vi "get binary trace.vi"(7 "error in (no error)":errorcluster, 9 "Trace Name (0:Trace1)":u16(ring) items=["Trace1", "Trace2", "Trace3", "Trace4", "Trace5", "Trace6", "Line1", "Line2"], 10 "VISA resource in":refnum<visa-resource-name>) -> (0 "error out":errorcluster, 1 "Stop frequency(Hz)":dbl format="%#_13g", 2 "Start frequency (Hz)":dbl format="%#_13g", 3 "VISA resource out":refnum<visa-resource-name>, 4 "Number of points":i32, 5 "Linear frequecny increment (Hz)":dbl format="%#_13g", 6 "Trace Array (1D)":dbl[](array[numeric]))   [LabVIEW 2016]
doc: "Get binary trace information from PSA screen, output start/stop/frequency, linear frequency increment, Y value 1D Array data."
panel:
  out "Waveform Graph":dbl[](graph)
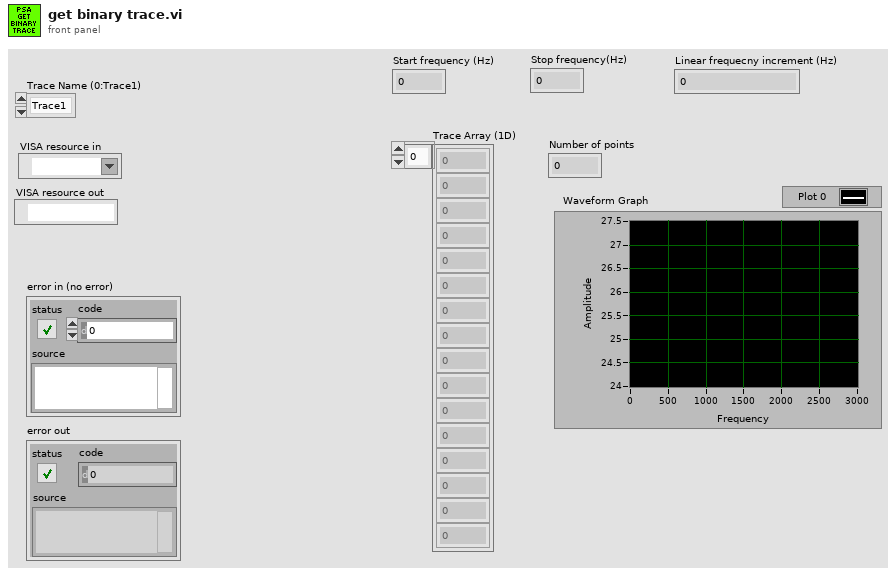
[diagram p1: front panel]
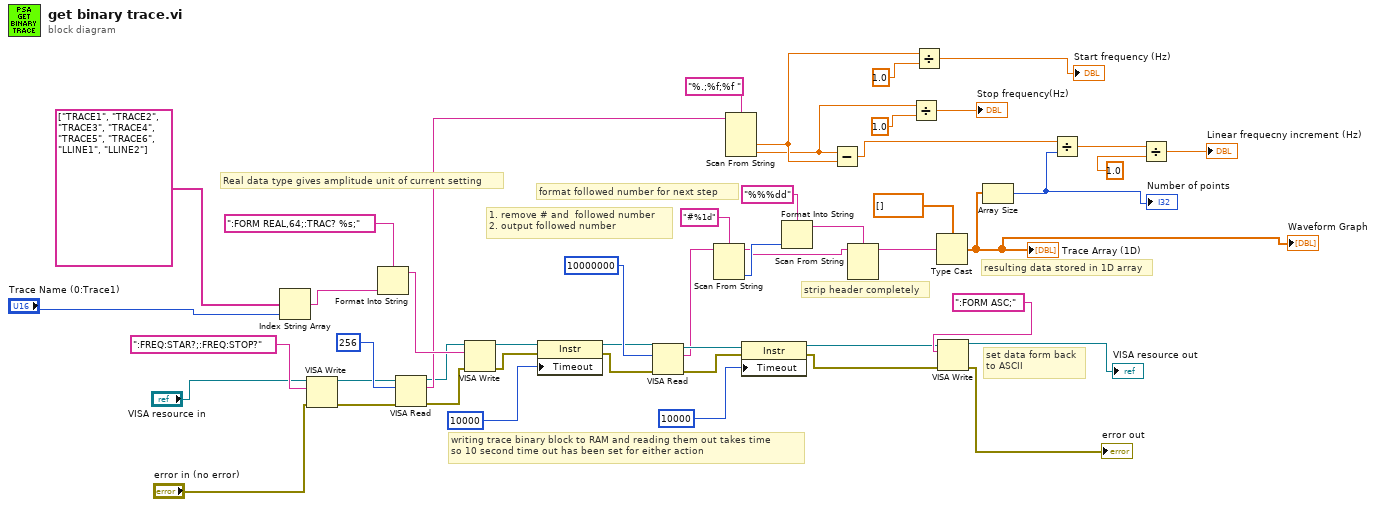
[diagram p0: block diagram]
diagram:
  # "set data form back\nto ASCII"
  # "writing trace binary block to RAM and reading them out takes time\nso 10 second time out has been set for either action"
  # "resulting data stored in 1D array"
  # "strip header completely"
  # "format followed number for next step"
  # "1. remove # and  followed number\n2. output followed number"
  # "Real data type gives amplitude unit of current setting"
  n1 = Index String Array(1:"Trace Name (0:Trace1)", 2:string[] ["TRACE1", "TRACE2", "TRACE3", "TRACE4", "TRACE5", "TRACE6", "LLINE1", "LLINE2"] ("string array")) -> (0:w46:string)  [unwired: 1 in]
  n2 = VISA Write(VISA resource name="VISA resource in", write buffer=":FREQ:STAR?;:FREQ:STOP?", error in (no error)="error in (no error)") -> (VISA resource name out=w27:refnum<visa-resource-name>, error out=w20:errorcluster)  [unwired: 1 out]
  n3 = Format Into String(format string=":FORM REAL,64;:TRAC? %s;", w46) -> (resulting string=w45:string)  [unwired: 2 in, 1 out]
  n4 = VISA Read(VISA resource name=w27, byte count=u32 256, error in (no error)=w20) -> (VISA resource name out=w12:refnum<visa-resource-name>, read buffer=w25:string, error out=w19:errorcluster)  [unwired: 1 out]
  n5 = VISA Write(VISA resource name=w12, write buffer=w45, error in (no error)=w19) -> (VISA resource name out=w43:refnum<visa-resource-name>, error out=w18:errorcluster)  [unwired: 1 out]
  n6 = property class="Instr"(reference=w43, error in=w18, "Timeout"=u32 10000 ("General Settings:Timeout Value")) -> (reference out=w41:refnum<visa-resource-name>, error out=w17:errorcluster)
  n7 = VISA Read(VISA resource name=w41, byte count=u32 10000000, error in (no error)=w17) -> (VISA resource name out=w39:refnum<visa-resource-name>, read buffer=w38:string, error out=w16:errorcluster)  [unwired: 1 out]
  n8 = Scan From String(format string="#%1d", input string=w38) -> (remaining string=w34:string, output 1=w36:i32)  [unwired: 3 in, 2 out]
  n9 = Scan From String(format string="%.;%f;%f ", input string=w25) -> (output 1=w11:dbl, output 2=w9:dbl)  [unwired: 4 in, 3 out]
  n10 = property class="Instr"(reference=w39, error in=w16, "Timeout"=u32 10000 ("General Settings:Timeout Value")) -> (reference out=w22:refnum<visa-resource-name>, error out=w15:errorcluster)
  n11 = Format Into String(format string="%%%dd", w36) -> (resulting string=w33:string)  [unwired: 2 in, 1 out]
  n12 = Subtract(x=w9, y=w11) -> (x-y=w24:dbl)
  n13 = Scan From String(format string=w33, input string=w34) -> (remaining string=w32:string)  [unwired: 4 in, 2 out]
  n14 = Divide(x=w9, y=1.0) -> (x/y=→"Stop frequency(Hz)":dbl)
  n15 = Divide(x=w11, y=1.0) -> (x/y=→"Start frequency (Hz)":dbl)
  n16 = Type Cast(type=dbl[] [], x=w32) -> (*(type *) &x=w1:dbl[])
  "Trace Array (1D)" <- w1
  "Waveform Graph" <- w1
  n17 = VISA Write(VISA resource name=w22, write buffer=":FORM ASC;", error in (no error)=w15) -> (VISA resource name out=→"VISA resource out":refnum<visa-resource-name>, error out=→"error out":errorcluster)  [unwired: 1 out]
  n18 = Array Size(array=w1) -> (size(s)=w6:i32)
  "Number of points" <- w6
  n19 = Divide(x=w24, y=w6) -> (x/y=w5:dbl)
  n20 = Divide(x=w5, y=1.0) -> (x/y=→"Linear frequecny increment (Hz)":dbl)
